vi "Map.vi"() -> ()   [LabVIEW 2020, in "Examples.lvlib"]
doc: "Example that showcases how to use Map by capitalizing the first character of strings."
uses:
  Examples.lvlib
  225e6126-9a79-4860-8837-1c7bd6ffe87f.vi
  Capitalize.vi
panel:
  out "Capitalized Strings":string[](array[string])
  in  "Strings":string[](array[string])=["test", "string", "word"]
  # "1) Take note of the existing strings in the Strings control. Add new ones if you would like.\n2) Run the VI.\n3) Note that the first character of the strings has been capitalized in Capitalized Strings.\n4) View the block diagram."
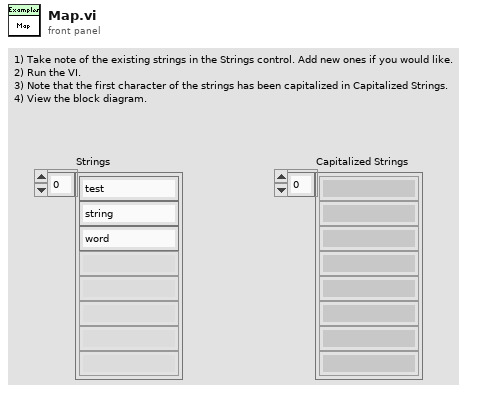
[diagram p1: front panel]
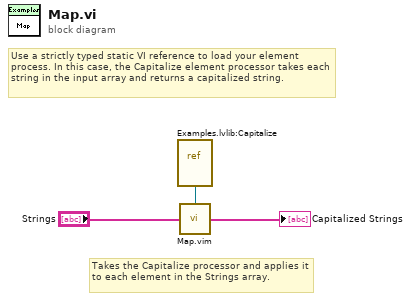
[diagram p0: block diagram]
diagram:
  # "Takes the Capitalize processor and applies it to each element in the Strings array."
  # "Use a strictly typed static VI reference to load your element process. In this case, the Capitalize element processor takes each string in the input array and returns a capitalized string."
  n1 = vi-ref "Examples.lvlib:Capitalize.vi"() -> (w3:refnum<vi>)
  n2 = call "Map.vim"("Processor"=w3, "Array"="Strings") -> ("Mapped Array"=→"Capitalized Strings":string[])  [unwired: 2 in]
